vi "ReadGlobal.vi"   [LabVIEW 2010]
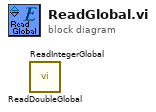
[diagram p0: block diagram]
diagram:
  n1 = call "ReadIntegerGlobal.vi"() -> ()  [unwired: 9 in, 3 out]
  n2 = call "ReadDoubleGlobal.vi"() -> ()  [unwired: 9 in, 3 out]
